vi "Excel Get Data ([i32]).vi"(0 "report in":refnum<class "NI_report.lvclass">, 5 "data type":i32[][](array[numeric]), 7 "start (-1, -1)":cluster{"row":i32, "column":i32}={"row"=-1, "column"=-1}, 9 "end (-1, -1)":cluster{"row":i32, "column":i32}={"row"=-1, "column"=-1}, 11 "error in (no error)":errorcluster, 12 "name (\"\")":string) -> (4 "report out":refnum<class "NI_report.lvclass">, 8 "data":i32[][](array[numeric]), 15 "error out":errorcluster)   [LabVIEW 2010, in "NI_Excel.lvclass"]
doc: "Retrieves data from the current worksheet. The data type you wire to the <B>data type</B> input determines the polymorphic instance to use."
uses:
  <vilib>/Utility/NIReport.llb/Excel/NI_Excel.lvclass
  <vilib>/Utility/NIReport.llb/NI_report.lvclass
  <vilib>/Utility/NIReport.llb/Excel/NI_Excel.lvclass/NI_Excel.ctl
  <vilib>/addons/_office/NI_ReportGenerationToolkit.lvlib
  <vilib>/Utility/NIReport.llb/NI_ReportGenerationCore.lvlib
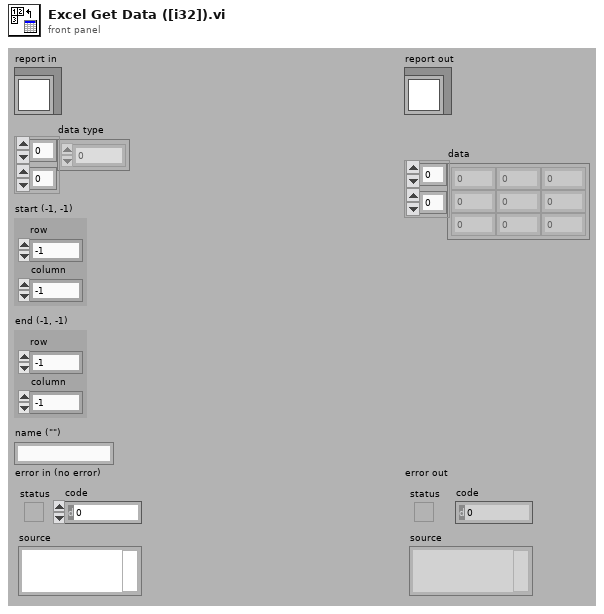
[diagram p1: front panel]
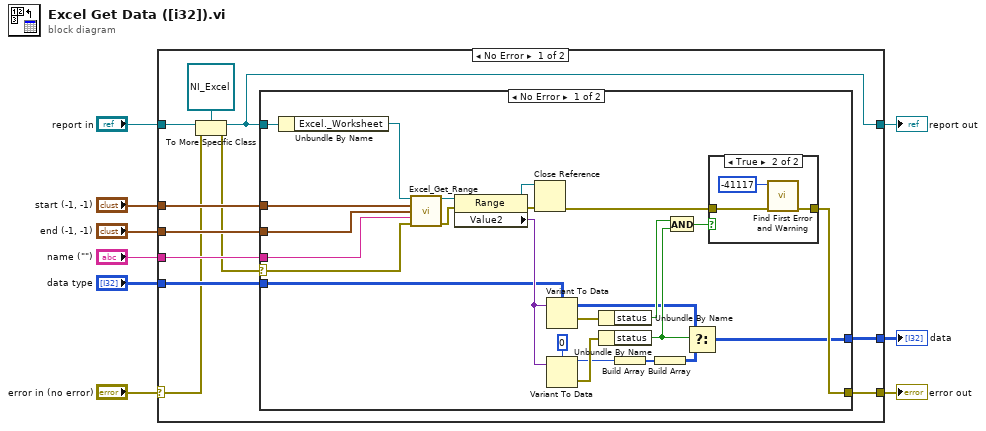
[diagram p0: block diagram]
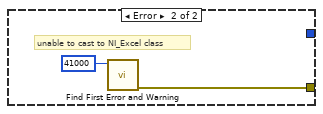
[diagram p3: hidden frame]
diagram:
  n1 = case shown="No Error" "error in (no error)" {
    selector: "error in (no error)" -> [w10 w53]
    tunnel: [w20 w53] -> w8
    tunnel: [w12 w52] -> w6
    tunnel: "report in" -> [w13 w52]
    tunnel: "start (-1, -1)" -> [w19 _]
    tunnel: "end (-1, -1)" -> [w18 _]
    tunnel: "name (\"\")" -> [w17 _]
    tunnel: "data type" -> [w16 _]
    tunnel: [w15 _] -> w1
    frame No Error {
      n2 = To More Specific Class(target class=refnum<class "NI_Excel.lvclass"> refnum ("report in"), reference=w13, error in=w10) -> (specific class reference=w12:refnum<class "NI_Excel.lvclass">, error out=w11:errorcluster)
      n3 = case shown="No Error" w11 {
        selector: w11 -> [w21 _]
        tunnel: [w29 w50] -> w20
        tunnel: w19 -> [w28 _]
        tunnel: w18 -> [w27 _]
        tunnel: w17 -> [w26 _]
        tunnel: w16 -> [w25 _]
        tunnel: [w23 _] -> w15
        tunnel: w12 -> [w22 _]
        frame No Error {
          n4 = Unbundle By Name(w22) -> ("Excel._Worksheet"=w24:refnum<k7>)
          n5 = call <vilib>:"Excel_Get_Range.vi"("Excel._Worksheet"=w24, "start"=w28, "end"=w27, "name"=w26, "error in (no error)"=w21) -> ("Range"=w42:refnum<k7>, "error out"=w43:errorcluster)  [unwired: 5 in, 4 out]
          n6 = property class="Range"(reference=w42, error in=w43) -> (reference out=w31:refnum<k7>, error out=w30:errorcluster, "Value2"=w32:variant)
          n7 = Close Reference(reference=w31, error in (no error)=w30) -> (error out=w40:errorcluster)
          n8 = Variant To Data(Variant=w32, type=w25) -> (error out=w44:errorcluster, data=w37:i32[][])  [unwired: 1 in]
          n9 = Variant To Data(Variant=w32, type=0) -> (error out=w45:errorcluster, data=w34:i32)  [unwired: 1 in]
          n10 = Unbundle By Name(w44) -> ("status"=w39:bool)
          n11 = Unbundle By Name(w45) -> ("status"=w38:bool)
          n12 = Build Array(w34) -> (w35:i32[])
          n13 = Build Array(w35) -> (w36:i32[][])
          n14 = And(x=w39, y=w38) -> (x .and. y?=w41:bool)
          n15 = Select(t=w37, s=w38, f=w36) -> (s? t:f=w23:i32[][])
          n16 = case shown="True" w41 {
            tunnel: w40 -> [w46 w48]
            tunnel: [w46 w47] -> w29
            frame False {
            }
            frame True {
              n17 = call <vilib>:"Find First Error and Warning.vi"("error in (no error)"=w48, "error code"=-41117) -> ("error out"=w47:errorcluster)  [unwired: 1 in, 4 out]
            }
          }
        }
        frame Error {
          # "unable to cast to NI_Excel class"
          n18 = call <vilib>:"Find First Error and Warning.vi"("error code"=41000) -> ("error out"=w50:errorcluster)  [unwired: 2 in, 4 out]
        }
      }
    }
    frame Error {
    }
  }
  "error out" <- w8
  "report out" <- w6
  "data" <- w1
